vi "Generate Schedule Status.vi"(8 "error in (no error)":errorcluster, 9 "Current Action":string, 10 "Monkey Status":T2=enum."Ongoing", 11 "Monkey in":refnum<class "Monkey.lvclass">) -> (0 "error out":errorcluster, 2 "Monkey Status Message":T1={"Monkey ID"="", "Monkey Status"=enum."Ongoing", "Scripts left"=0, "ETA"="", "Current Action"="", "Report from previous RUNs"="", "Skipped RUNs"=refnum}, 3 "Monkey out":refnum<class "Monkey.lvclass">)   [LabVIEW 2020, in "Monkey.lvlib" / "Monkey.lvclass"]
uses:
  Monkey.lvclass
  C:/Users/marco/Documents/GitHub_Lab/TALOS/talos/Father of all uServices/Father of all uServices/Father of all uServices.lvclass
  C:/Users/marco/Documents/GitHub_Lab/TALOS/talos/Ancestor/Ancestor/Ancestor.lvclass
  Run Utilities/TypeDefs/Monkey Status.ctl
  Run Utilities/TypeDefs/Messages/Monkey Status Message.ctl
  Run Utilities/Schedule/Schedule.lvclass
  Monkey.lvclass/Monkey.ctl
  Ancestor/Ancestor/Ancestor.lvclass/Ancestor.ctl
  Father of all uServices/Father of all uServices/Father of all uServices.lvclass/Father of all uServices.ctl
  Ancestor/Ancestor/Read ID.vi
  Support VIs/Generate Error.vi
  FGV/Error Memory/Get Error Description.vi
  Support VIs/Get PC name.vi
  Support VIs/Get Class Name.vi
  <vilib>/Utility/error.llb/Clear Errors.vi
  FGV/Error Memory/Error Memory Core.vi
  <vilib>/AdvancedString/Delimited String to 1D String Array.vi
  Support VIs/Circus Root Path.vi
  FGV/Error Memory/Error Crt Lvl checker.vi
  FGV/Error Memory/Error Memory Core.vi/40c8088d-b597-4017-91af-faa98e00292e.vi
  FGV/Error Memory/Error Memory Core.vi/d4a3ab98-063c-4e44-b43d-fbdcfe6c2be2.vi
  Support VIs/Global Memory.vi
  <vilib>/Utility/LVClass/Get LV Class Name.vi
  Support VIs/Is in Packed Library.vi
  Support VIs/TALOS Root path.vi
  Support VIs/Read CSV worksheet.vi
  Support VIs/Global Constants.vi
  <vilib>/Utility/error.llb/General Error Handler.vi
  Support VIs/Error Log.vi
  Ancestor/Ancestor/Ancestor.lvclass
  <vilib>/Comparison/Equal/Equal Functor/Equal Functor.lvclass
  Run Utilities/Run Block/Run Block.lvclass
  Run Utilities/Run Utilities.lvlib
  Father of all uServices/Father of all uServices/Father of all uServices.lvclass
  TALOS.lvlib
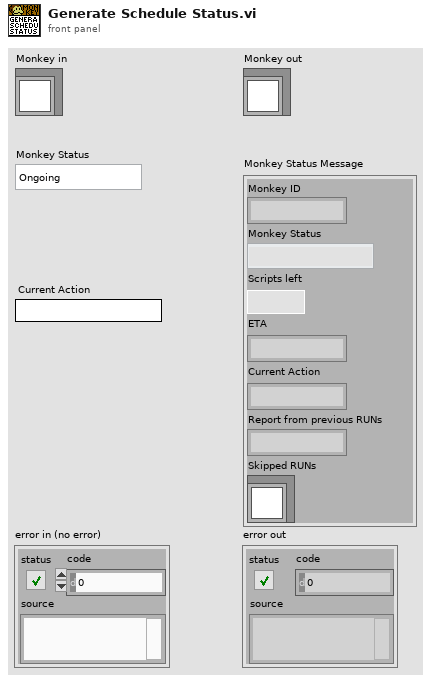
[diagram p1: front panel]
types:
  T1 = typedef "TALOS.lvlib/Run Utilities.lvlib/Monkey Status Message.ctl" = cluster{"Monkey ID":string, "Monkey Status":T2, "Scripts left":u32, "ETA":string, "Current Action":string, "Report from previous RUNs":string, "Skipped RUNs":refnum<class "Schedule.lvclass">}
  T2 = typedef "TALOS.lvlib/Run Utilities.lvlib/Monkey Status.ctl" = enum16{"Init", "Paused", "Ongoing", "Stopped", "Finished (no errors)", "Finished (with errors)"}
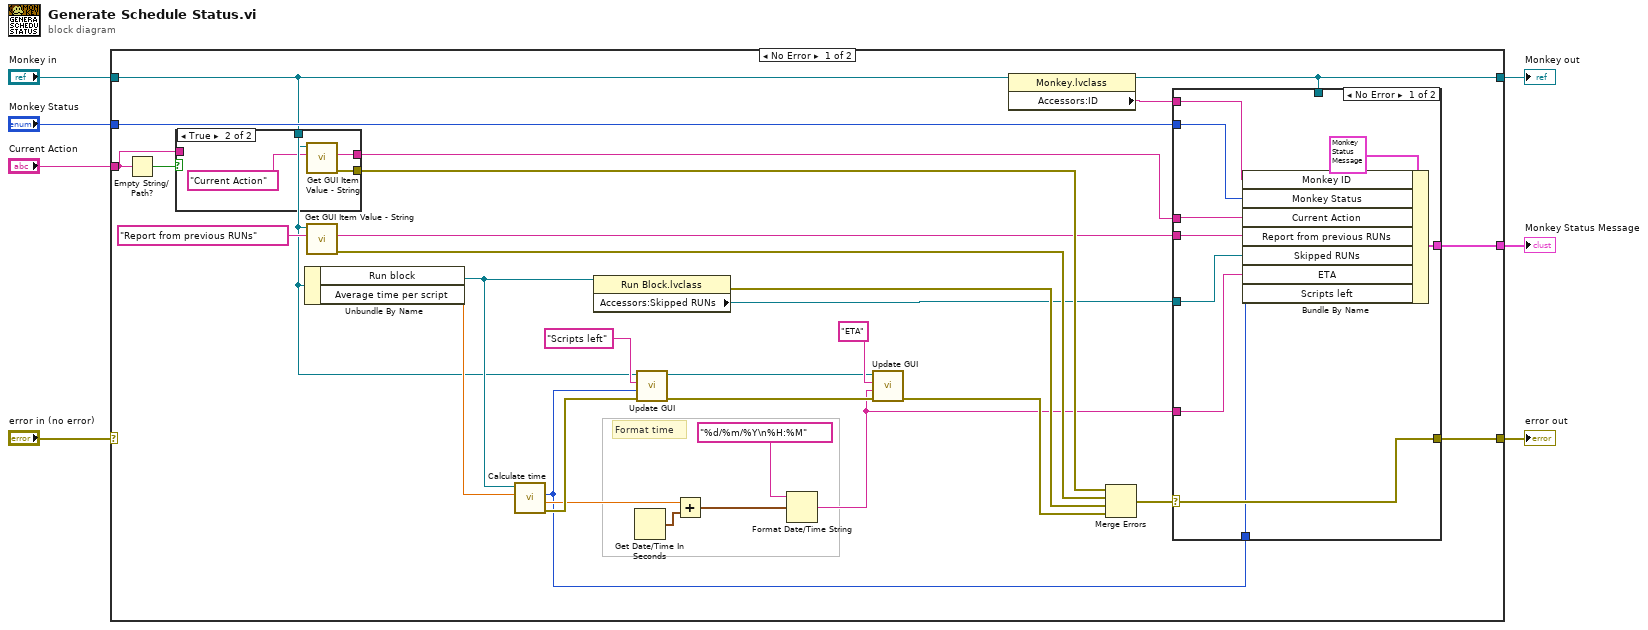
[diagram p0: block diagram]
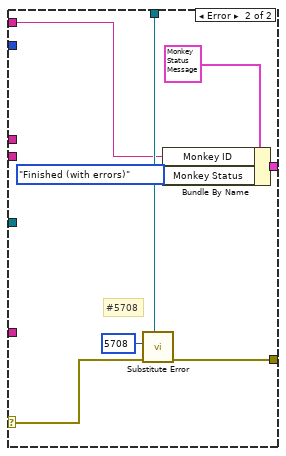
[diagram p3: hidden frame]
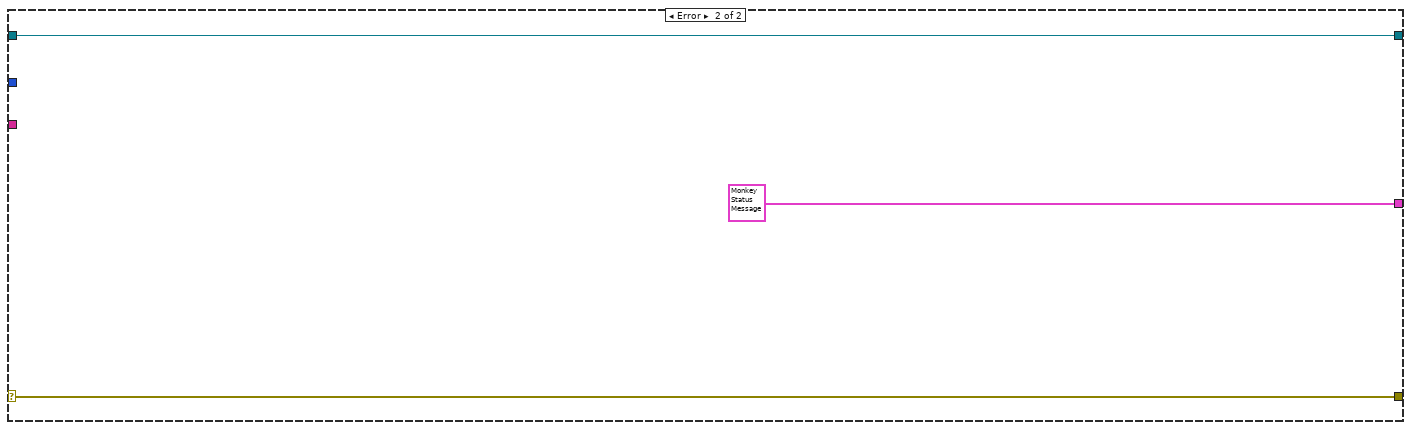
[diagram p4: hidden frame]
diagram:
  n1 = case shown="No Error" "error in (no error)" {
    selector: "error in (no error)" -> [_ w63]
    tunnel: [w31 w63] -> w6
    tunnel: "Monkey in" -> [w13 w62]
    tunnel: [w26 w62] -> w4
    tunnel: [w30 T1 {"Monkey ID"="", "Monkey Status"=enum."Ongoing", "Scripts left"=0, "ETA"="", "Current Action"="", "Report from previous RUNs"="", "Skipped RUNs"=refnum} ("Monkey Status Message")] -> w2
    tunnel: "Monkey Status" -> [w29 _]
    tunnel: "Current Action" -> [w8 _]
    frame No Error {
      # "Format time"
      n2 = Empty String/Path?(string/path=w8) -> (empty?=w9:bool)
      n3 = case shown="True" w9 {
        tunnel: [_ w42] -> w37
        tunnel: [w38 w40] -> w32
        tunnel: w13 -> [_ w39]
        tunnel: w8 -> [w38 _]
        frame False {
        }
        frame True {
          n4 = call "Get GUI Item Value - String.vi"("FP Item Name"="Current Action", "uService Template in"=w39) -> ("error out"=w42:errorcluster, "Value"=w40:string)  [unwired: 7 in, 1 out]
        }
      }
      n5 = Unbundle By Name(w13) -> ("Run block"=w14:refnum<class "Run Block.lvclass">, "Average time per script"=w15:dbl)
      n6 = call "Get GUI Item Value - String.vi"("FP Item Name"="Report from previous RUNs", "uService Template in"=w13) -> ("error out"=w36:errorcluster, "Value"=w33:string)  [unwired: 7 in, 1 out]
      n7 = call-dynamic "Calculate time.vi"("Average time"=w15, "Run Block in"=w14) -> ("error out"=w24:errorcluster, "Time"=w18:dbl, "Number of scripts"=w10:u32)  [unwired: 6 in, 1 out]
      n8 = property class="Run Block.lvclass"(reference=w14) -> (error out=w28:errorcluster, "Accessors:Skipped RUNs"=w27:refnum<class "Schedule.lvclass">)  [unwired: 1 in, 1 out]
      n9 = Get Date/Time In Seconds() -> (seconds since 1Jan1904=w21:timestamp)
      n10 = call "Update GUI.vi"("error in (no error)"=w24, "Data"=w10, "GUI Item Name"="Scripts left", "uService Template in"=w13) -> ("error out"=w16:errorcluster, "uService Template out"=w17:refnum<class "Monkey.lvclass">)  [unwired: 6 in]
      n11 = Add(x=w18, y=w21) -> (x+y=w19:timestamp)
      n12 = Format Date/Time String(time format string (%c)="%d/%m/%Y\n%H:%M", seconds (now)=w19) -> (date/time string=w11:string)  [unwired: 1 in]
      n13 = call "Update GUI.vi"("error in (no error)"=w16, "Data"=w11, "GUI Item Name"="ETA", "uService Template in"=w17) -> ("error out"=w12:errorcluster)  [unwired: 6 in, 1 out]
      n14 = property class="Monkey.lvclass"(reference=w13) -> (reference out=w26:refnum<class "Monkey.lvclass">, "Accessors:ID"=w25:string)  [unwired: 1 in, 1 out]
      n15 = Merge Errors(w37, w36, w28, w12) -> (w34:errorcluster)
      n16 = case shown="No Error" w34 {
        selector: w34 -> [w49 w60]
        tunnel: w27 -> [w50 _]
        tunnel: w33 -> [w51 _]
        tunnel: w32 -> [w52 _]
        tunnel: [w49 w59] -> w31
        tunnel: [w47 w55] -> w30
        tunnel: w26 -> [_ w58]
        tunnel: w29 -> [w48 _]
        tunnel: w25 -> [w45 w54]
        tunnel: w11 -> [w44 _]
        tunnel: w10 -> [w43 _]
        frame No Error {
          n17 = Bundle By Name(cluster=T1 {"Monkey ID"="", "Monkey Status"=enum."Ongoing", "Scripts left"=0, "ETA"="", "Current Action"="", "Report from previous RUNs"="", "Skipped RUNs"=refnum} ("Monkey Status Message"), "Monkey ID"=w45, "Monkey Status"=w48, "Current Action"=w52, "Report from previous RUNs"=w51, "Skipped RUNs"=w50, "ETA"=w44, "Scripts left"=w43) -> (w47:T1)
        }
        frame Error {
          # "#5708"
          n18 = call "Substitute Error.vi"("LabVIEW Object"=w58, "error in (no error)"=w60, "Error Code"=5708) -> ("error out"=w59:errorcluster)  [unwired: 8 in]
          n19 = Bundle By Name(cluster=T1 {"Monkey ID"="", "Monkey Status"=enum."Ongoing", "Scripts left"=0, "ETA"="", "Current Action"="", "Report from previous RUNs"="", "Skipped RUNs"=refnum} ("Monkey Status Message"), "Monkey ID"=w54, "Monkey Status"=Monkey_Status."Finished (with errors)") -> (w55:T1)
        }
      }
    }
    frame Error {
    }
  }
  "Monkey out" <- w4
  "error out" <- w6
  "Monkey Status Message" <- w2
